vi "NI VeriStand - Clear All Faults.vi"(8 "error in (no error)":errorcluster, 11 "ChannelFault in":T1) -> (0 "error out":errorcluster, 3 "ChannelFault out":T1)   [LabVIEW 2020, in "NI_VS ChannelFault ExecutionAPI.lvlib"]
doc: "Clears all active faults on the target."
uses:
  <vilib>/NI VeriStand/Execution/ChannelFaultManager/NI_VS ChannelFault ExecutionAPI.lvlib
  <vilib>/NI VeriStand/Execution/ChannelFaultManager/ChannelFaultAPI.ctl
  NationalInstruments.VeriStand.ClientAPI
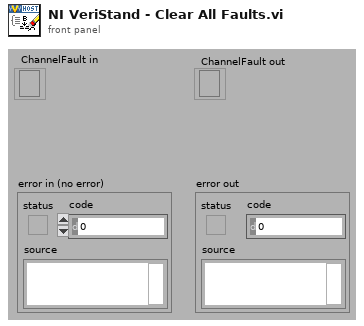
[diagram p1: front panel]
types:
  T1 = typedef "NI_VS ChannelFault ExecutionAPI.lvlib/ChannelFaultAPI.ctl" = refnum<k24>
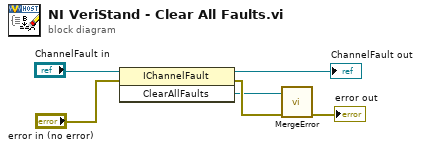
[diagram p0: block diagram]
diagram:
  n1 = invoke class="IChannelFault" method="ClearAllFaults"(reference="ChannelFault in", error in="error in (no error)") -> (reference out=→"ChannelFault out":T1, error out=w4:errorcluster, "ClearAllFaults"=w3:refnum<k24>)  [unwired: 1 in]
  n2 = call <vilib>:"MergeError.vi"("error in (no error)"=w4, "Error"=w3) -> ("error out"=→"error out":errorcluster)  [unwired: 9 out]
